vi "niScope Initiate Digitizing Process.vi"(8 "error in":errorcluster, 11 "niScope in":T1={"channel cfg"=[], "sessions"=[], "multi cards"=FALSE, "channels"=0, "type"=enum."n/a", "memory [B/chn]"=0, "ext. clock [Hz]"=0.0, "samples count"=0, "use streaming"=FALSE, "proc setup"={"packet size [smpl]"=0, "current timeout [s]"=0.0, "blk2blk timeout [s]"=0.0, "event time"=timestamp(0 s since 1904-01-01), "temp sampl T [s]"=0.0, "data queue"=refnum, "stop notifier"=refnum, "proc ref"=refnum}, "sample width [B]"=0, "ranges [V]"=[], "trigger setup"={"coupling"=1, "level [V]"=0.0, "slope"=0, "mode"=enum."Immediate"}, "fs [Hz]"=0.0, "bitres [bit]"=0} {"trigger setup"."level [V]" format="%.2f"; "trigger setup"."coupling" items=["AC"=0, "DC"=1, "HF Reject"=3, "LF Reject"=4, "AC Plus HF Reject"=1001]; "channel cfg"."Range [Vpk]" min=0.0; "channel cfg"."Channel" min=0}) -> (0 "error out":errorcluster, 3 "niScope out":T1={"channel cfg"=[], "sessions"=[], "multi cards"=FALSE, "channels"=0, "type"=enum."n/a", "memory [B/chn]"=0, "ext. clock [Hz]"=0.0, "samples count"=0, "use streaming"=FALSE, "proc setup"={"packet size [smpl]"=0, "current timeout [s]"=0.0, "blk2blk timeout [s]"=0.0, "event time"=timestamp(0 s since 1904-01-01), "temp sampl T [s]"=0.0, "data queue"=refnum, "stop notifier"=refnum, "proc ref"=refnum}, "sample width [B]"=0, "ranges [V]"=[], "trigger setup"={"coupling"=1, "level [V]"=0.0, "slope"=0, "mode"=enum."Immediate"}, "fs [Hz]"=0.0, "bitres [bit]"=0} {"trigger setup"."level [V]" format="%.2f"; "trigger setup"."coupling" items=["AC"=0, "DC"=1, "HF Reject"=3, "LF Reject"=4, "AC Plus HF Reject"=1001]; "channel cfg"."Range [Vpk]" min=0.0; "channel cfg"."Channel" min=0})   [LabVIEW 2018, in "niScope Virtual Digitizer.lvlib"]
doc: "Initiates acquisition for both single shot and streaming modes. It creates data queue and starts digitizing process which runs on background. If succeds the process immediatelly starts digitizing (depending on the trigger settings) and filling the queue with data. So this VI must be immediatelly followed by fetch loop that takes out data from the queue!"
uses:
  niScope Virtual Digitizer.lvlib
  niScope Session.ctl
  niScope Virtual Channel Config.ctl
  niScope Virtual Channel Mode.ctl
  niScope Virtual Channel Input Z.ctl
  niScope Virtual Channel Coupling.ctl
  niScope Type.ctl
  niScope Digitizing Process Options.ctl
  niScope Data Packet.ctl
  niScope Trigger Setup.ctl
  <instrlib>/niScope/Controls/niScope trigger coupling.ctl
  <instrlib>/niScope/Controls/niScope trigger slope.ctl
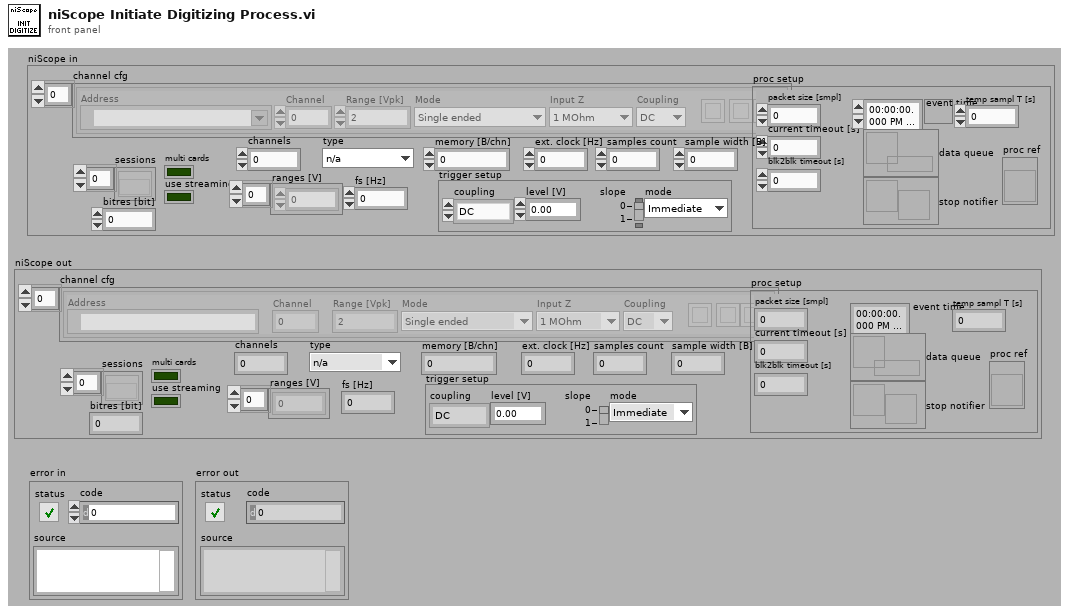
[diagram p1: front panel]
types:
  T1 = typedef "niScope Virtual Digitizer.lvlib/niScope Session.ctl" = cluster{"channel cfg":T2[], "sessions":refnum<k20>[], "multi cards":bool, "channels":i32, "type":T6, "memory [B/chn]":i32, "ext. clock [Hz]":dbl, "samples count":i64, "use streaming":bool, "proc setup":T7, "sample width [B]":i32, "ranges [V]":dbl[], "trigger setup":T8, "fs [Hz]":dbl, "bitres [bit]":i32}
  T2 = typedef "niScope Virtual Digitizer.lvlib/niScope Virtual Channel Config.ctl" = cluster{"Address":refnum<k15>, "Channel":i32, "Mode":T3, "Input Z":T4, "Coupling":T5, "Range [Vpk]":dbl, "btn clr":bool, "btn up":bool, "btn down":bool}
  T3 = typedef "niScope Virtual Digitizer.lvlib/niScope Virtual Channel Mode.ctl" = enum16{"Single ended", "Unbal. differential", "Differential"}
  T4 = typedef "niScope Virtual Digitizer.lvlib/niScope Virtual Channel Input Z.ctl" = enum16{"1 MOhm", "50 Ohm"}
  T5 = typedef "niScope Virtual Digitizer.lvlib/niScope Virtual Channel Coupling.ctl" = enum16{"AC", "DC", "GND"}
  T6 = typedef "niScope Virtual Digitizer.lvlib/niScope Type.ctl" = enum16{"n/a", "5922"}
  T7 = typedef "niScope Virtual Digitizer.lvlib/niScope Digitizing Process Options.ctl" = cluster{"packet size [smpl]":i64, "current timeout [s]":dbl, "blk2blk timeout [s]":dbl, "event time":timestamp, "temp sampl T [s]":dbl, "data queue":refnum<queue>, "stop notifier":refnum<notifier>, "proc ref":refnum<vi>}
  T8 = typedef "niScope Virtual Digitizer.lvlib/niScope Trigger Setup.ctl" = cluster{"coupling":T9, "level [V]":dbl, "slope":T10, "mode":enum16{"Immediate", "External", "Level"}}
  T9 = typedef "niScope trigger coupling.ctl" = u16
  T10 = typedef "niScope trigger slope.ctl" = i32
  T11 = typedef "niScope Virtual Digitizer.lvlib/niScope Data Packet.ctl" = cluster{"int32":i32[][], "card buffer [%]":dbl, "all done?":bool, "offset [smpl]":i64, "sampling?":bool, "queue buffer [%]":dbl, "int16":i16[][], "is int16?":bool, "count [smpl]":i32, "valid?":bool}
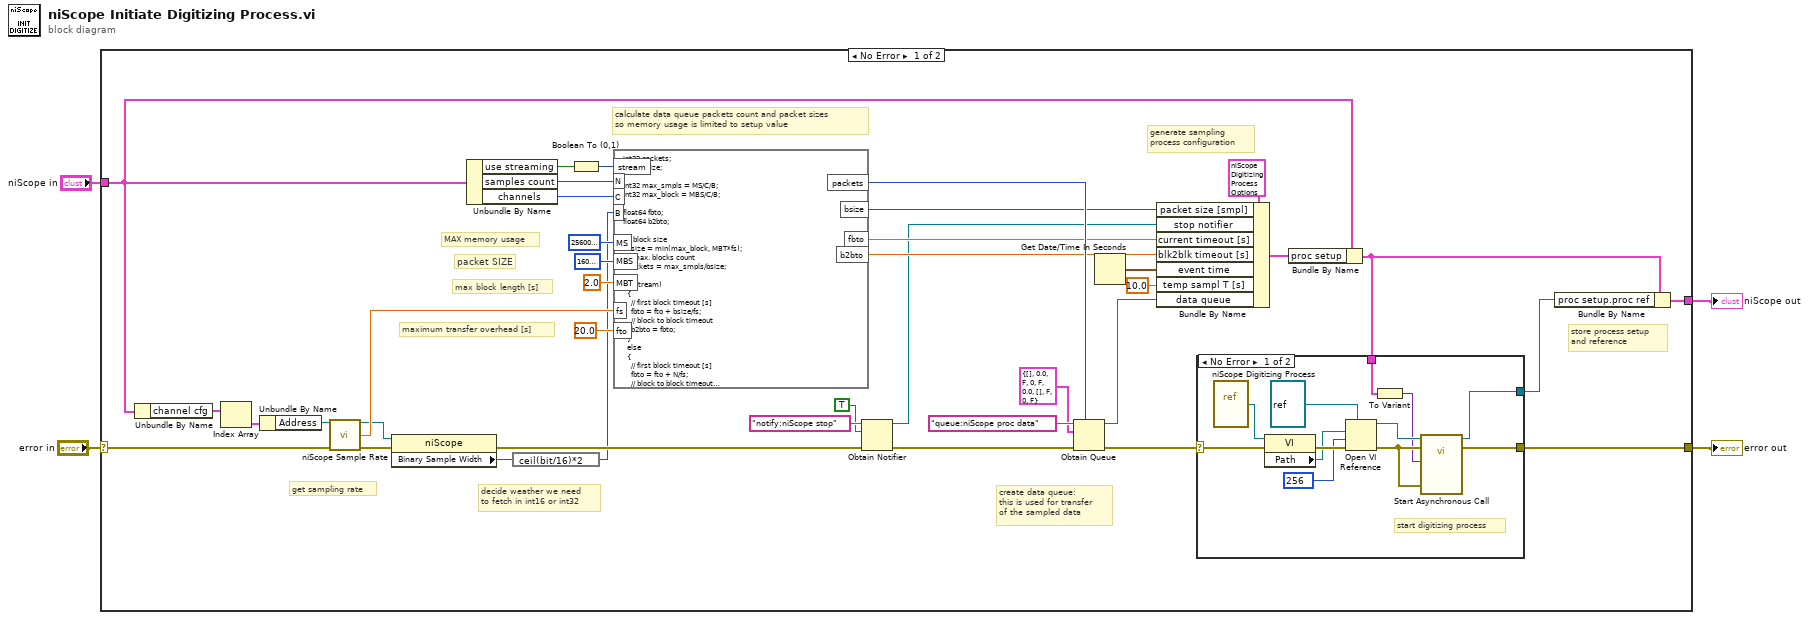
[diagram p0: block diagram]
diagram:
  n1 = case shown="No Error" "error in" {
    selector: "error in" -> [w19 w58]
    tunnel: [w11 w58] -> w4
    tunnel: "niScope in" -> [w14 w57]
    tunnel: [w23 w57] -> w2
    frame No Error {
      # "decide weather we need\nto fetch in int16 or int32"
      # "store process setup\nand reference"
      # "maximum transfer overhead [s]"
      # "generate sampling\nprocess configuration"
      # "calculate data queue packets count and packet sizes\nso memory usage is limited to setup value"
      # "get sampling rate"
      # "max block length [s]"
      # "packet SIZE"
      # "MAX memory usage"
      # "create data queue:\nthis is used for transfer\nof the sampled data"
      n2 = Unbundle By Name(w14) -> ("channel cfg"=w35:T2[])
      n3 = Index Array(array=w35) -> (element=w34:T2)  [unwired: 1 in]
      n4 = Unbundle By Name(w34) -> ("Address"=w33:refnum<k15>)
      n5 = call <instrlib>:"niScope Sample Rate.vi"("instrument handle"=w33, "error in"=w19) -> ("instrument handle out"=w9:refnum<k15>, "actual sample rate"=w32:dbl, "error out"=w10:errorcluster)  [unwired: 11 in]
      n6 = property class="niScope"(reference=w9, error in=w10) -> (error out=w7:errorcluster, "Binary Sample Width"=w8:i32)  [unwired: 1 out]
      n7 = Unbundle By Name(w14) -> ("use streaming"=w41:bool, "samples count"=w39:i64, "channels"=w38:i32)
      n8 = expression code="ceil(bit/16)*2"(w8) -> (w6:i32)
      n9 = Boolean To (0,1)(Boolean=w41) -> (0, 1=w40:i16)
      n10 = formula code="int32 packets;\nint32 bsize;\n\nint32 max_smpls = MS/C/B;\nint32 max_block = MBS/C/B;\n\nfloat64 fbto;\nfloat64 b2bto;\n\n  // block size\n  bsize = min(max_block, MBT*fs);\n  // max. blocks count\n  packets = max_smpls/bsize;\n\n  if(stream)\n  {\n    // first block timeout [s]\n    fbto = fto + bsize/fs;\n    // block to block timeout\n    b2bto = fbto;\n  }\n  else\n  {\n    // first block timeout [s]\n    fbto = fto + N/fs;\n    // block to block timeout\n    b2bto = fto + bsize/fs;\n  }"("stream"=w40, "N"=w39, "C"=w38, "MS"=256000000 ("y"), "MBS"=16000000 ("y"), "fs"=w32, "MBT"=2.0 ("input variable"), "fto"=20.0 ("input variable"), "B"=w6) -> ("packets"=w30:i32, "bsize"=w29:i32, "fbto"=w26:dbl, "b2bto"=w24:dbl)
      n11 = Obtain Notifier(name (unnamed)="notify:niScope stop", notification data type=TRUE, error in (no error)=w7) -> (notifier out=w15:refnum<notifier>, error out=w17:errorcluster)  [unwired: 1 in, 1 out]
      n12 = Obtain Queue(max queue size (-1, unlimited)=w30, name (unnamed)="queue:niScope proc data", element data type=T11 {"int32"=[], "card buffer [%]"=0.0, "all done?"=FALSE, "offset [smpl]"=0, "sampling?"=FALSE, "queue buffer [%]"=0.0, "int16"=[], "is int16?"=FALSE, "count [smpl]"=0, "valid?"=FALSE} ("niScope packet"), error in (no error)=w17) -> (queue out=w21:refnum<queue>, error out=w28:errorcluster)  [unwired: 1 in, 1 out]
      n13 = Get Date/Time In Seconds() -> (seconds since 1Jan1904=w25:timestamp)
      n14 = Bundle By Name(cluster=T7 {"packet size [smpl]"=0, "current timeout [s]"=0.0, "blk2blk timeout [s]"=0.0, "event time"=timestamp(0 s since 1904-01-01), "temp sampl T [s]"=0.0, "data queue"=refnum, "stop notifier"=refnum, "proc ref"=refnum} ("setup"), "packet size [smpl]"=w29, "stop notifier"=w15, "current timeout [s]"=w26, "blk2blk timeout [s]"=w24, "event time"=w25, "temp sampl T [s]"=10.0, "data queue"=w21) -> (w13:T7)
      n15 = Bundle By Name(cluster=w14, "proc setup"=w13) -> (w5:T1)
      n16 = case shown="No Error" w28 {
        selector: w28 -> [w46 w56]
        tunnel: [w47 w56] -> w11
        tunnel: [w45 _] -> w12
        tunnel: w5 -> [w44 _]
        frame No Error {
          # "start digitizing process"
          n17 = vi-ref "niScope Digitizing Process.vi"() -> (w54:refnum<vi>)
          n18 = property class="VI"(reference=w54, error in=w46) -> (error out=w53:errorcluster, "Path"=w51:path)  [unwired: 1 out]
          n19 = Open VI Reference(type specifier VI Refnum (for type only)=refnum<vi> refnum, vi path=w51, options=256, error in (no error)=w53) -> (vi reference=w55:refnum<vi>, error out=w52:errorcluster)  [unwired: 2 in]
          n20 = To Variant(anything=w44) -> (Variant=w48:variant)
          n21 = call-by-ref "Start Asynchronous Call"(reference=w55, error in=w52, "error in"=w52, "niScope session"=w48) -> (reference out=w45:refnum<vi>, error out=w47:errorcluster)  [unwired: 8 in, 2 out]
        }
        frame Error {
        }
      }
      n22 = Bundle By Name(cluster=w5, "proc setup.proc ref"=w12) -> (w23:T1)
    }
    frame Error {
    }
  }
  "error out" <- w4
  "niScope out" <- w2
